vi "PPSSelfTest.vi"(8 "error in (no error)":errorcluster, 11 "IT-M3904D in":refnum<class "IT-M3904D.lvclass">) -> (0 "error out":errorcluster, 2 "Self-Test Result Message":string, 3 "IT-M3904D out":refnum<class "IT-M3904D.lvclass">)   [LabVIEW 2023, in "HardwareAbstractionLayer_LVOOP.lvlib" / "IT-M3904D.lvclass"]
uses:
  IT-M3904D.lvclass
  PowerSupply.lvclass
  <instrlib>/IT-M3900D/IT-M3900D.lvlib
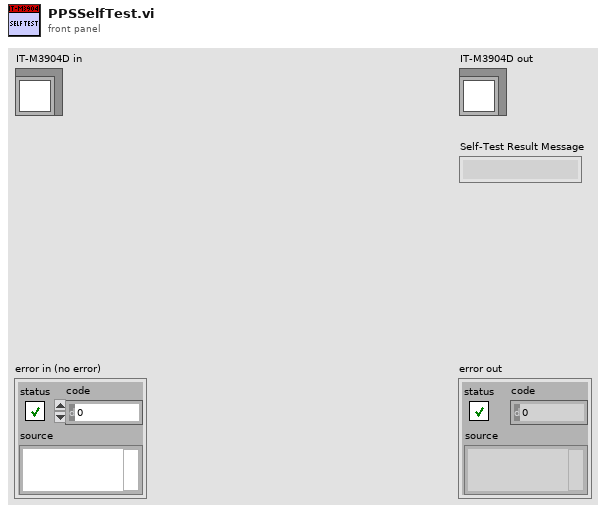
[diagram p1: front panel]
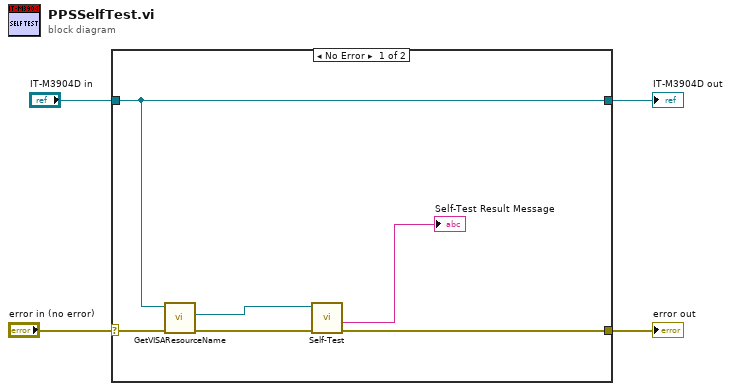
[diagram p0: block diagram]
diagram:
  n1 = case shown="No Error" "error in (no error)" {
    selector: "error in (no error)" -> [w10 w12]
    tunnel: "IT-M3904D in" -> [w9 w11]
    tunnel: [w7 w12] -> w2
    tunnel: [w9 w11] -> w1
    frame No Error {
      n2 = call "GetVISAResourceName.vi"("error in (no error)"=w10, "object in"=w9) -> ("error out"=w8:errorcluster, "VISA resource name"=w6:refnum<visa-resource-name>)  [unwired: 7 in, 1 out]
      n3 = call <instrlib>:"Self-Test.vi"("error in"=w8, "VISA resource name"=w6) -> ("error out"=w7:errorcluster, "Self-Test Result Message"=→"Self-Test Result Message":string)  [unwired: 6 in, 2 out]
    }
    frame Error {
    }
  }
  "error out" <- w2
  "IT-M3904D out" <- w1
